vi "Open Waveform Sessions.vi"(8 "error in":errorcluster, 11 "Async State Vars":T1) -> (0 "error out":errorcluster, 3 "Async State Vars out":T1)   [LabVIEW 2020, in "Waveform-Processing-Custom-Device Engine.lvlib"]
uses:
  Waveform-Processing-Custom-Device Engine.lvlib
  Types/AsyncStateVariables.ctl
  <vilib>/NI VeriStand/Custom Device Waveform API/Single Waveform Read (DBL)/Single Waveform Read (DBL).lvclass
  <vilib>/NI VeriStand/Custom Device Waveform API/Single Waveform Write (DBL)/Single Waveform Write (DBL).lvclass
  <vilib>/NI VeriStand/Custom Device API/Waveform Data Reference.ctl
  <vilib>/NI/NIVS Inline Async API/_Data Access Engine/Data Access Engine/Types/Write.DVR.ctl
  <vilib>/NI/NIVS Inline Async API/_Data Access Engine/Access Type Classes/Write/Write.lvclass
  <vilib>/NI/NIVS Inline Async API/_Data Access Engine/Data Access Engine/Types/Read.DVR.ctl
  <vilib>/NI/NIVS Inline Async API/_Data Access Engine/Access Type Classes/Read/Read.lvclass
  <vilib>/NI VeriStand/Custom Device Waveform API/Single Waveform Read (DBL)/NI VeriStand - Open Single Waveform Read Session (DBL).vi
  <vilib>/NI VeriStand/Custom Device Waveform API/Single Waveform Write (DBL)/NI VeriStand - Open Single Waveform Write Session (DBL).vi
  <vilib>/NI VeriStand/Custom Device Waveform API/NI_VS Custom Device Waveform API.lvlib
  <vilib>/NI VeriStand/Custom Device API/Custom Device API.lvlib
  <vilib>/NI/NIVS Inline Async API/_Data Access Engine/Data Access Engine/Data Access Engine.lvclass
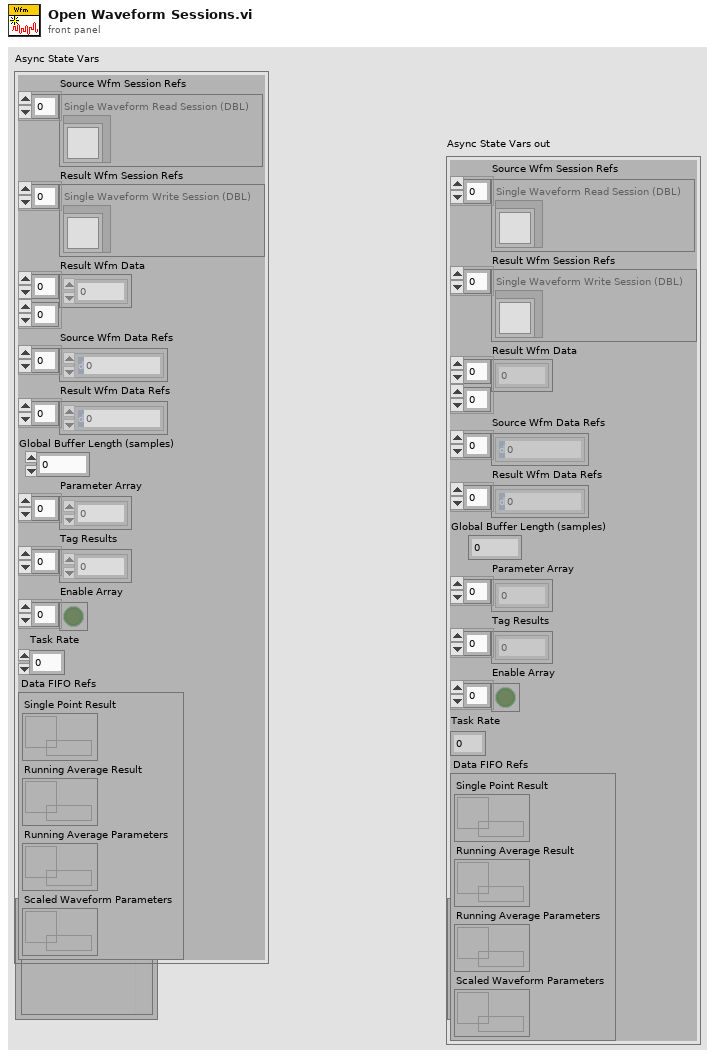
[diagram p1: front panel]
types:
  T1 = typedef "Waveform-Processing-Custom-Device Engine.lvlib/AsyncStateVariables.ctl" = cluster{"Source Wfm Session Refs":refnum<class "Single Waveform Read (DBL).lvclass">[], "Result Wfm Session Refs":refnum<class "Single Waveform Write (DBL).lvclass">[], "Result Wfm Data":dbl[][], "Source Wfm Data Refs":T2[], "Result Wfm Data Refs":T2[], "Global Buffer Length (samples)":dbl, "Parameter Array":dbl[], "Tag Results":dbl[], "Enable Array":bool[], "Task Rate":dbl, "Data FIFO Refs":cluster{"Single Point Result":T3, "Running Average Result":T3, "Running Average Parameters":T4, "Scaled Waveform Parameters":T4}}
  T2 = typedef "Custom Device API.lvlib/Waveform Data Reference.ctl" = i32
  T3 = typedef "Data Access Engine.lvlib/Data Access Engine.lvclass/Write.DVR.ctl" = refnum<data-value>
  T4 = typedef "Data Access Engine.lvlib/Data Access Engine.lvclass/Read.DVR.ctl" = refnum<data-value>
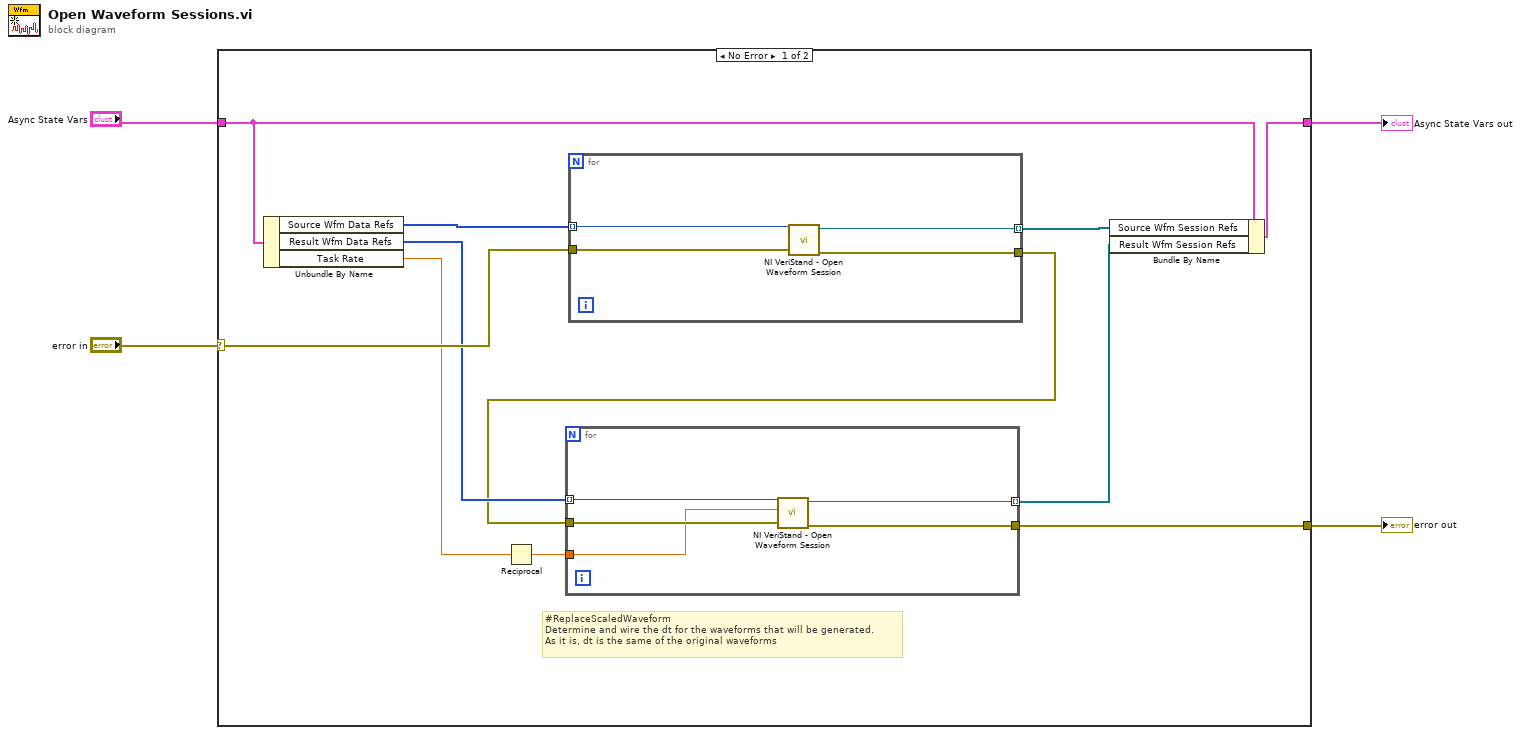
[diagram p0: block diagram]
diagram:
  n1 = case shown="No Error" "error in" {
    selector: "error in" -> [w12 w26]
    tunnel: [w7 w26] -> w3
    tunnel: "Async State Vars" -> [w11 w25]
    tunnel: [w13 w25] -> w1
    frame No Error {
      # "#ReplaceScaledWaveform \nDetermine and wire the dt for the waveforms that will be generated.\nAs it is, dt is the same of the original waveforms"
      n2 = Unbundle By Name(w11) -> ("Source Wfm Data Refs"=w15:T2[], "Result Wfm Data Refs"=w10:T2[], "Task Rate"=w6:dbl)
      n3 = Reciprocal(x=w6) -> (1/x=w5:dbl)
      n4 = for {
        tunnel: [w24] -> w9
        tunnel: w15 -> [w22] mode=indexing
        tunnel: [w23] -> w14 mode=indexing
        tunnel: w12 -> [w21]
        n5 = call-poly <vilib>:"NI VeriStand - Open Waveform Session.vi"("error in (no error)"=w21, "DBL Waveform Data Reference"=w22) -> ("error out"=w24:errorcluster, "Single Waveform Read Session (DBL)"=w23:refnum<class "Single Waveform Read (DBL).lvclass">)  [unwired: 8 in]
      }
      n6 = for {
        tunnel: [w20] -> w7
        tunnel: w10 -> [w18] mode=indexing
        tunnel: [w19] -> w8 mode=indexing
        tunnel: w9 -> [w17]
        tunnel: w5 -> [w16]
        n7 = call-poly <vilib>:"NI VeriStand - Open Waveform Session.vi"("error in (no error)"=w17, "dt"=w16, "DBL Waveform Data Reference"=w18) -> ("error out"=w20:errorcluster, "Single Waveform Write Session (DBL)"=w19:refnum<class "Single Waveform Write (DBL).lvclass">)  [unwired: 7 in]
      }
      n8 = Bundle By Name(cluster=w11, "Source Wfm Session Refs"=w14, "Result Wfm Session Refs"=w8) -> (w13:T1)
    }
    frame Error {
    }
  }
  "error out" <- w3
  "Async State Vars out" <- w1
